vi "fetch_and_translate_trigger.vi"(8 "error in (no error)":errorcluster, 11 "ScanHeadMH100729FPGA in":refnum<class "ScanHeadMH100729FPGA.lvclass">) -> (0 "error out":errorcluster, 1 "sender TLC type":T1=enum."ImagingMode", 2 "internal trigger":T2, 3 "ScanHeadMH100729FPGA out":refnum<class "ScanHeadMH100729FPGA.lvclass">)   [LabVIEW 2010, in "ScanHeadMH100729FPGA.lvclass"]
uses:
  ScanHeadMH100729FPGA.lvclass
  internal_trigger_enum.ctl
  common/enumerations/top-level_component_type_enum.ctl
  GenericScanHead/GenericScanHead/trigger_enum.ctl
  GenericScanHead/GenericScanHead/GenericScanHead.lvclass
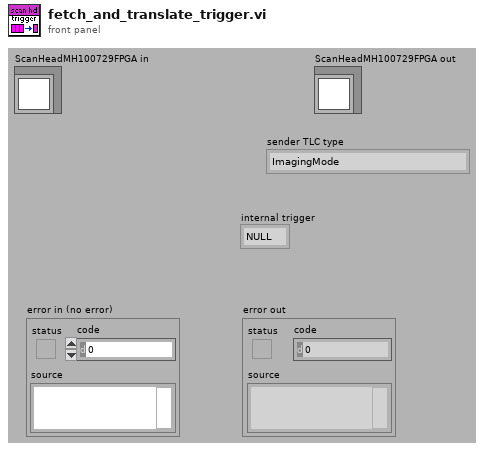
[diagram p1: front panel]
types:
  T1 = typedef "top-level_component_type_enum.ctl" = enum16{"undefined", "ImagingMode", "ScanHead", "DAQ", "ImageAssembler", "Display", "DataCollection", "Analyser", "Stimulator", "ExperimentController", "Instrument", "Stage"}
  T2 = typedef "ScanHeadMH100729FPGA.lvclass/internal_trigger_enum.ctl" = enum16{"NULL", "initialise", "terminate", "start scanning", "stop scanning", "update", "fetch trajectory"}
  T3 = typedef "GenericScanHead.lvclass/trigger_enum.ctl" = enum16{"NULL", "fetch trajectory", "generate trajectory", "change run mode", "update modifiers"}
  T4 = typedef "GenericToplevelComponent.lvclass/common_trigger_enum.ctl" = enum16{"NULL", "initialise", "terminate", "fetch command", "fetch data", "attach observer", "register as observer", "detach observer", "acknowledge", "start", "stop", "sweep started", "sweep finished", "experiment started", "experiment stopped"}
  T5 = typedef "trigger_type_enum.ctl" = enum8{"external", "internal", "common"}
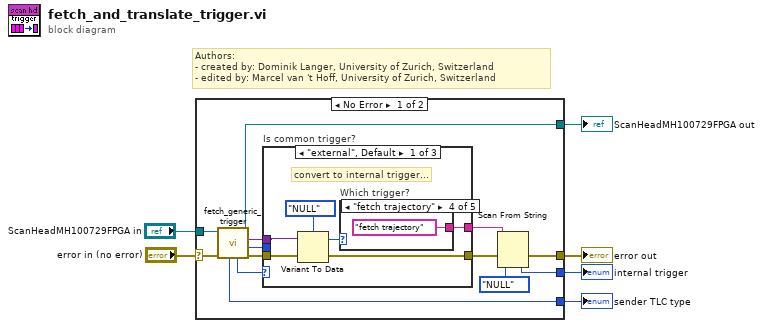
[diagram p0: block diagram]
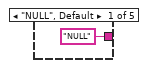
[diagram p2: hidden frame]
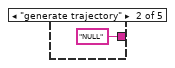
[diagram p3: hidden frame]
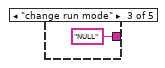
[diagram p4: hidden frame]
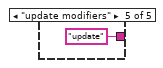
[diagram p5: hidden frame]
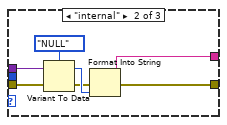
[diagram p6: hidden frame]
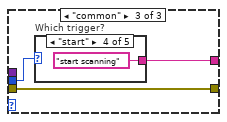
[diagram p7: hidden frame]
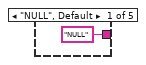
[diagram p8: hidden frame]
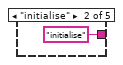
[diagram p9: hidden frame]
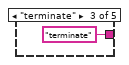
[diagram p10: hidden frame]
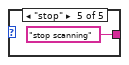
[diagram p11: hidden frame]
diagram:
  # "Authors: \n- created by: Dominik Langer, University of Zurich, Switzerland\n- edited by: Marcel van 't Hoff, University of Zurich, Switzerland"
  n1 = case shown="No Error" "error in (no error)" {
    selector: "error in (no error)" -> [w19 w47]
    tunnel: [w10 w47] -> w5
    tunnel: [w16 w46] -> w3
    tunnel: "ScanHeadMH100729FPGA in" -> [w17 w46]
    tunnel: [w8 _] -> w1
    tunnel: [w12 _] -> w2
    frame No Error {
      n2 = call-dynamic "fetch_generic_trigger.vi"("error in (no error)"=w19, "GenericToplevelComponent in"=w17) -> ("error out"=w18:errorcluster, "common trigger"=w13:T4, "trigger"=w14:variant, "GenericToplevelComponent out"=w16:refnum<class "ScanHeadMH100729FPGA.lvclass">, "trigger type"=w15:T5, "sender TLC type"=w12:T1)  [unwired: 3 in, 1 out]
      n3 = case "Is common trigger?" shown="\"external\", Default" w15 {
        tunnel: [w25 w31 w40] -> w9
        tunnel: w18 -> [w24 w37 w40]
        tunnel: w14 -> [w23 w36 _]
        tunnel: w13 -> [_ _ w39]
        tunnel: [w20 w33 w38] -> w7
        frame "external", Default {
          # "convert to internal trigger..."
          n4 = Variant To Data(error in=w24, Variant=w23, type=trigger_enum."NULL" ("trigger")) -> (error out=w25:errorcluster, data=w22:T3)
          n5 = case "Which trigger?" shown="\"fetch trajectory\"" w22 {
            tunnel: ["NULL" "NULL" "NULL" "fetch trajectory" "update"] -> w20
            frame "NULL", Default {
            }
            frame "generate trajectory" {
            }
            frame "change run mode" {
            }
            frame "fetch trajectory" {
            }
            frame "update modifiers" {
            }
          }
        }
        frame "internal" {
          n6 = Variant To Data(error in=w37, Variant=w36, type=internal_trigger_enum."NULL" ("internal trigger")) -> (error out=w32:errorcluster, data=w34:T2)
          n7 = Format Into String(error in=w32, w34) -> (resulting string=w33:string, error out=w31:errorcluster)  [unwired: 2 in]
        }
        frame "common" {
          n8 = case "Which trigger?" shown="\"start\"" w39 {
            tunnel: ["NULL" ("input string") "initialise" ("input string") "terminate" ("input string") "start scanning" ("input string") "stop scanning" ("input string")] -> w38
            frame "NULL", Default {
            }
            frame "initialise" {
            }
            frame "terminate" {
            }
            frame "start" {
            }
            frame "stop" {
            }
          }
        }
      }
      n9 = Scan From String(input string=w7, error in=w9, default 1=internal_trigger_enum."NULL" ("internal trigger")) -> (error out=w10:errorcluster, output 1=w8:T2)  [unwired: 2 in, 2 out]
    }
    frame Error {
    }
  }
  "error out" <- w5
  "internal trigger" <- w1
  "ScanHeadMH100729FPGA out" <- w3
  "sender TLC type" <- w2
